vi "SendRequestToFAMM.vi"(7 "FAMM-function":T1, 8 "error in (no error)":errorcluster, 9 "Data":variant, 10 "Source":string, 11 "Gserver in":refnum<class "Gserver.lvclass">) -> (0 "error out":errorcluster, 3 "Gserver out":refnum<class "Gserver.lvclass">)   [LabVIEW 2020, in "Sgraph_lib_V1.lvlib" / "Gserver.lvclass"]
doc: "Andre Koelewijn, 17 jan 2021\n\nSend a message to the FAMM service"
uses:
  Gserver.lvclass
  FAMM/controls/typedef-functions.ctl
  FAMM/controls/typedef_FAMM_Query.ctl
  Gserver.lvclass/Gserver.ctl
  Builds/Sgraph_lib_V1.lvlib
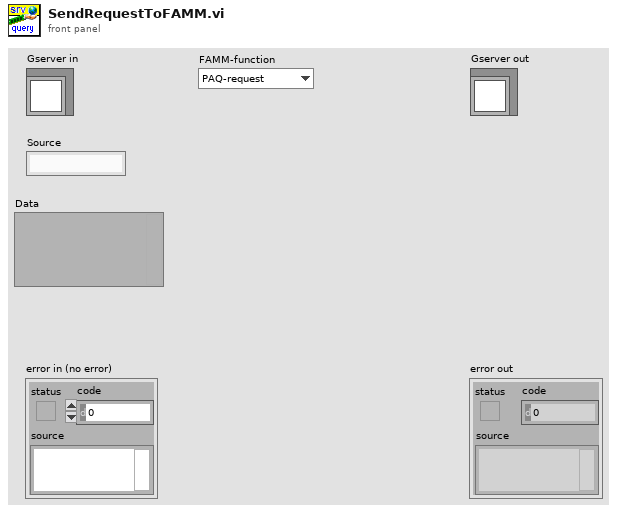
[diagram p1: front panel]
types:
  T1 = typedef "Sgraph_lib_V1.lvlib/typedef-functions.ctl" = enum16{"PAQ-request", "PAQ-taglist-request", "WAQ-request", "EAQ-request", "TAG-based-request", "PAQ-MemoryMap", "Update-TAG-property", "Exit-FAMM"}
  T2 = typedef "typedef_FAMM_Query.ctl" = cluster{"Time Stamp":timestamp, "FAMM-function":T1, "Source":string, "Data":variant}
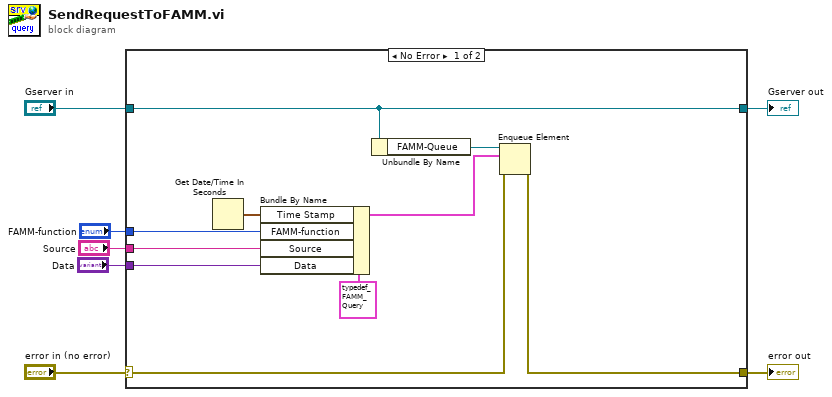
[diagram p0: block diagram]
diagram:
  n1 = case shown="No Error" "error in (no error)" {
    selector: "error in (no error)" -> [w13 w19]
    tunnel: [w12 w19] -> w6
    tunnel: [w17 w18] -> w4
    tunnel: "Gserver in" -> [w17 w18]
    tunnel: "FAMM-function" -> [w10 _]
    tunnel: "Source" -> [w9 _]
    tunnel: "Data" -> [w8 _]
    frame No Error {
      n2 = Get Date/Time In Seconds() -> (seconds since 1Jan1904=w11:timestamp)
      n3 = Bundle By Name(cluster=T2 {"Time Stamp"=timestamp(0 s since 1904-01-01), "FAMM-function"=enum."PAQ-request", "Source"="", "Data"=variant} ("element"), "Time Stamp"=w11, "FAMM-function"=w10, "Source"=w9, "Data"=w8) -> (w14:T2)
      n4 = Unbundle By Name(w17) -> ("FAMM-Queue"=w16:refnum<queue>)
      n5 = Enqueue Element(queue=w16, element=w14, error in (no error)=w13) -> (error out=w12:errorcluster)  [unwired: 1 in, 2 out]
    }
    frame Error {
    }
  }
  "error out" <- w6
  "Gserver out" <- w4
